vi "RSZVB Set Sweep Number Of Points.vi"(8 "error in (no error)":errorcluster {"code" format="%.0x"}, 9 "Number Of Points (201)":i32=201, 10 "Channel (1)":i32=1, 11 "VISA session":refnum<visa-resource-name>) -> (0 "error out":errorcluster {"code" format="%.0x"}, 3 "dup VISA session":refnum<visa-resource-name>)   [LabVIEW 2015]
doc: "This VI defines the total number of measurement points per sweep.\n\nRemote-control command(s):\n[SENSe<Ch>:]SWEep:POINts"
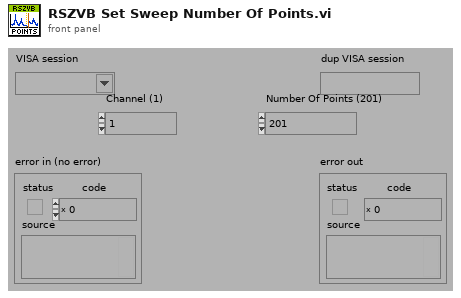
[diagram p1: front panel]
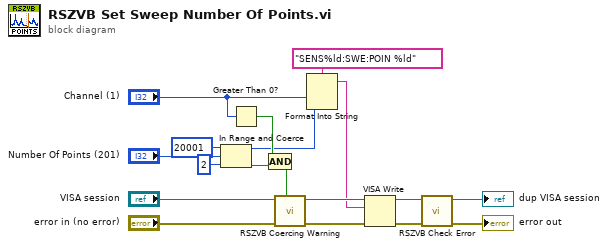
[diagram p0: block diagram]
diagram:
  n1 = In Range and Coerce(upper limit=20001, x="Number Of Points (201)", lower limit=2) -> (coerced(x)=w1:i32, In Range?=w4:bool)
  n2 = Greater Than 0?(x="Channel (1)") -> (x > 0?=w6:bool)
  n3 = Compound Arithmetic op=AND(w6, w4) -> (w13:bool)
  n4 = call "RSZVB Coercing Warning.vi"("In Range?"=w13, "error in (no error)"="error in (no error)", "VISA session"="VISA session") -> ("error out"=w16:errorcluster, "dup VISA session"=w17:refnum<visa-resource-name>)  [unwired: 7 in]
  n5 = Format Into String(format string="SENS%ld:SWE:POIN %ld", "Channel (1)", w1) -> (resulting string=w12:string)  [unwired: 2 in, 1 out]
  n6 = VISA Write(VISA resource name=w17, write buffer=w12, error in (no error)=w16) -> (VISA resource name out=w14:refnum<visa-resource-name>, error out=w15:errorcluster)  [unwired: 1 out]
  n7 = call "RSZVB Check Error.vi"("error in (no error)"=w15, "VISA session"=w14) -> ("error out"=→"error out":errorcluster, "dup VISA session"=→"dup VISA session":refnum<visa-resource-name>)  [unwired: 8 in]
